vi "Test Starting while Running Dose Not Replace View.vi"(8 "error in (no error)":errorcluster, 11 "View Test In":refnum<class "View Dev Test.lvclass">) -> (0 "error out":errorcluster, 3 "View Test Out":refnum<class "View Dev Test.lvclass">)   [LabVIEW 2020, in "View Dev Test.lvclass"]
uses:
  View Dev Test.lvclass
  C:/Program Files (x86)/National Instruments/LabVIEW 2020/vi.lib/Astemes/LUnit/Test Case.lvclass
  source/Framework/Process/Process.lvclass/Process.ctl
  source/Framework/Synchronous Request Callback/Synchronous Request Callback.lvclass/Synchronous Request Callback.ctl
  source/Framework/View/View.lvclass/View.ctl
  <vilib>/Astemes/LUnit/Test Case.lvclass/Test Case.ctl
  459629c3-7219-46df-a51b-9a0b5a9dd135.vi
  source/Framework/Process/Protected/Messaging/Request Message.vi
  source/Framework/Process/Public/Lifecycle/Get Lifecycle State.vi
  <vilib>/Astemes/LUnit/Append Pass Result.vi
  <vilib>/Astemes/LUnit/Append Fail Result.vi
  <vilib>/Astemes/LUnit/Describe Comparison.vi
  <vilib>/Astemes/LUnit/Compare Variants.vi
  source/Framework/Process/Private/SubVIs/Handle Debug Data.vi
  source/Framework/Process/Private/SubVIs/Enqueue Request Message.vi
  source/Framework/Synchronous Request Callback/Create.vi
  <vilib>/Utility/error.llb/Clear Errors.vi
  <vilib>/Astemes/LUnit/Variant to string.vi
  source/Framework/Logging/Log Debug.vi
  <vilib>/AdvancedString/1D String Array to Delimited String.vi
  <vilib>/Utility/High Resolution Relative Seconds.vi
  source/Framework/View/View.lvclass
  C:/git/astemes-triarc-framework/source/Framework/Process/Process.lvclass
  source/Framework/Synchronous Request Callback/Synchronous Request Callback.lvclass
  C:/git/astemes-triarc-framework/source/Framework/Callback/Callback.lvclass
  source/Framework/Process/Process.lvclass
  C:/git/astemes-triarc-framework/source/Framework/Logging/Logging.lvclass
  <vilib>/Utility/error.llb/Error Cluster From Error Code.vi
  source/Framework/Process/Public/Read Name.vi
  source/Framework/Process/Private/SubVIs/Wait for Response Message.vi
  <vilib>/Utility/Data Type/Get Type Information.vi
  <vilib>/Utility/LVClass/Get LV Class Name.vi
  source/Framework/Callback/Callback.lvclass
  source/Framework/Logging/Logging.lvclass
  View Dev Test.lvclass/View Dev Test.ctl
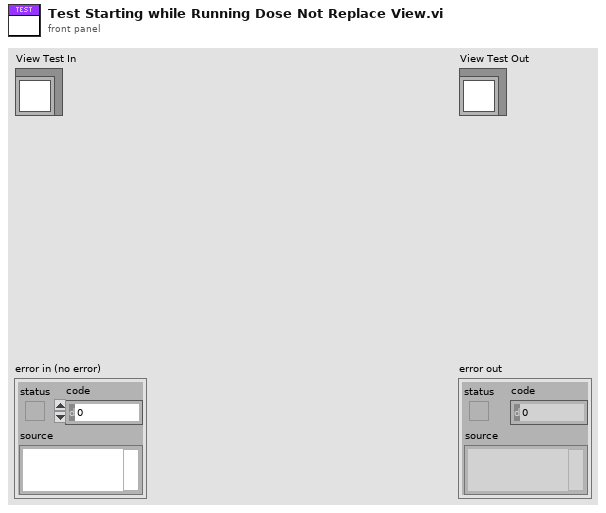
[diagram p1: front panel]
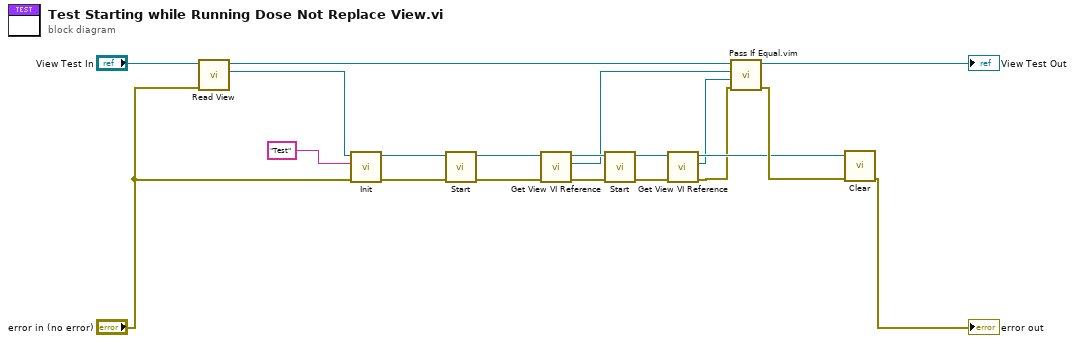
[diagram p0: block diagram]
diagram:
  n1 = call "Read View.vi"("error in (no error)"="error in (no error)", "View Test In"="View Test In") -> ("View"=w19:refnum<class "View.lvclass">, "View Test Out"=w20:refnum<class "View Dev Test.lvclass">)  [unwired: 7 in, 1 out]
  n2 = call-dynamic "Init.vi"("error in (no error)"="error in (no error)", "Name"="Test", "View In"=w19) -> ("error out"=w14:errorcluster, "View Out"=w9:refnum<class "View.lvclass">)  [unwired: 7 in]
  n3 = call "Start.vi"("error in (no error)"=w14, "Process In"=w9) -> ("error out"=w10:errorcluster, "Process Out"=w8:refnum<class "View.lvclass">)  [unwired: 7 in, 1 out]
  n4 = call "Get View VI Reference.vi"("error in (no error)"=w10, "View In"=w8) -> ("error out"=w7:errorcluster, "View VI Reference"=w1:refnum<vi>, "View Out"=w13:refnum<class "View.lvclass">)  [unwired: 7 in]
  n5 = call "Start.vi"("error in (no error)"=w7, "Process In"=w13) -> ("error out"=w5:errorcluster, "Process Out"=w6:refnum<class "View.lvclass">)  [unwired: 7 in, 1 out]
  n6 = call "Get View VI Reference.vi"("error in (no error)"=w5, "View In"=w6) -> ("error out"=w3:errorcluster, "View VI Reference"=w2:refnum<vi>, "View Out"=w4:refnum<class "View.lvclass">)  [unwired: 7 in]
  n7 = call "Pass If Equal.vim"("error in (no error)"=w3, "Actual"=w2, "Expected"=w1, "LUnit Test Case In"=w20) -> ("error out"=w11:errorcluster, "LUnit Test Case Out"=→"View Test Out":refnum<class "View Dev Test.lvclass">)  [unwired: 6 in]
  n8 = call-dynamic "Clear.vi"("error in (no error)"=w11, "View In"=w4) -> ("error out"=→"error out":errorcluster)  [unwired: 9 in]
